vi "LinearFilter_Execute_OLD.vi"(6 "Samples":i32=3 min=1, 7 "Filter Type":T1(ring), 8 "SamplePeriod":dbl=0.02 format="%13.5f", 9 "TimeConstant":dbl=0.02 format="%13.5f", 10 "Enable":bool=TRUE, 11 "Input":dbl format="%13.5p") -> (1 "Output":dbl format="%13.5p", 3 "Out LINEAR_FILTER":T2 {"Outputs" format="%13.5g"; "Inputs" format="%13.5g"; "OutputGains" format="%13.5g"; "InputGains" format="%13.5g"})   [LabVIEW 2019, in "Trajectory_Library.lvlib"]
doc: "This is a LabVIEW \"convience\" function that combines the various subVI for a linear filter into a single subVI. This subVI creates and executes the linear filter. The filter can be dynamically enabled and disabled. When the filter is disabled, the input is transfered directly to the output. Bumpless transfer is provided when enabling the filter. Bumpless transfer is NOT provided when disabling the filter. The output value jumps directly to the current input value. The filter type and filter constants can also be changed dynamically. When the filter contstants are changed, the output may jump to the current input value when the internal buffers are reset to the current input value.\n\nInputs:\n - FilterType - An enumerated value used to select the type of filter to be cofigured. The possible values are:\n - Moving Average - Specify the \"sample\" input.\n - Low pass 1st order Butterworth filter\n - Low pass 2nd order Butterworth filter\n - High pass 1st order Butterworth filter\n - High pass 2nd order Butterworth filter\n - Input - Input value to be filtered (Required) \n - Enable - Boolean indicating filtering should be performed (Default = True)\n - TimeConstant - Filtering time constant seconds. Used for all types except Moving \n Average (Default = 0.020) \n - SamplePeriod - Execution period seconds. Used for all types except Moving Average. \n (Default = 0.020)\n - Samples - Number of samples for the moving average filter. (Default = 3)\n\nOutputs:\n - OutLinearFilter - Current value of the LinearFilter data structure.\n - Output - Current output value."
uses:
  Trajectory_Library.lvlib
  TypeDef/LINEAR_FILTER.ctl
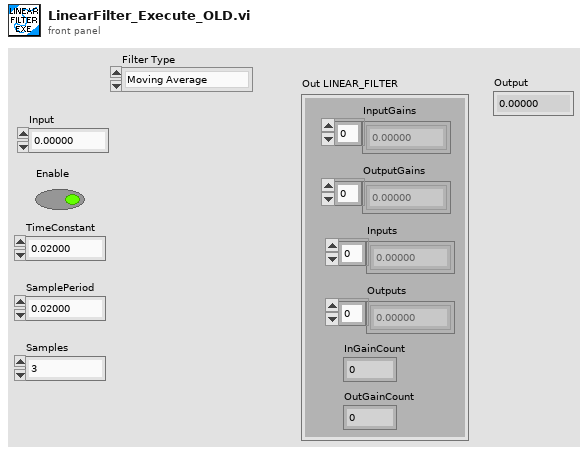
[diagram p1: front panel]
types:
  T1 = enum16{"Moving Average", "Low Pass 1st Order Butterworth", "Low Pass 2nd Order Butterworth", "High Pass 1st Order Butterworth", "High Pass 2nd Order Butterworth"}
  T2 = typedef "Trajectory_Library.lvlib/LINEAR_FILTER.ctl" = cluster{"InputGains":dbl[], "OutputGains":dbl[], "Inputs":dbl[], "Outputs":dbl[], "InGainCount":i32, "OutGainCount":i32}
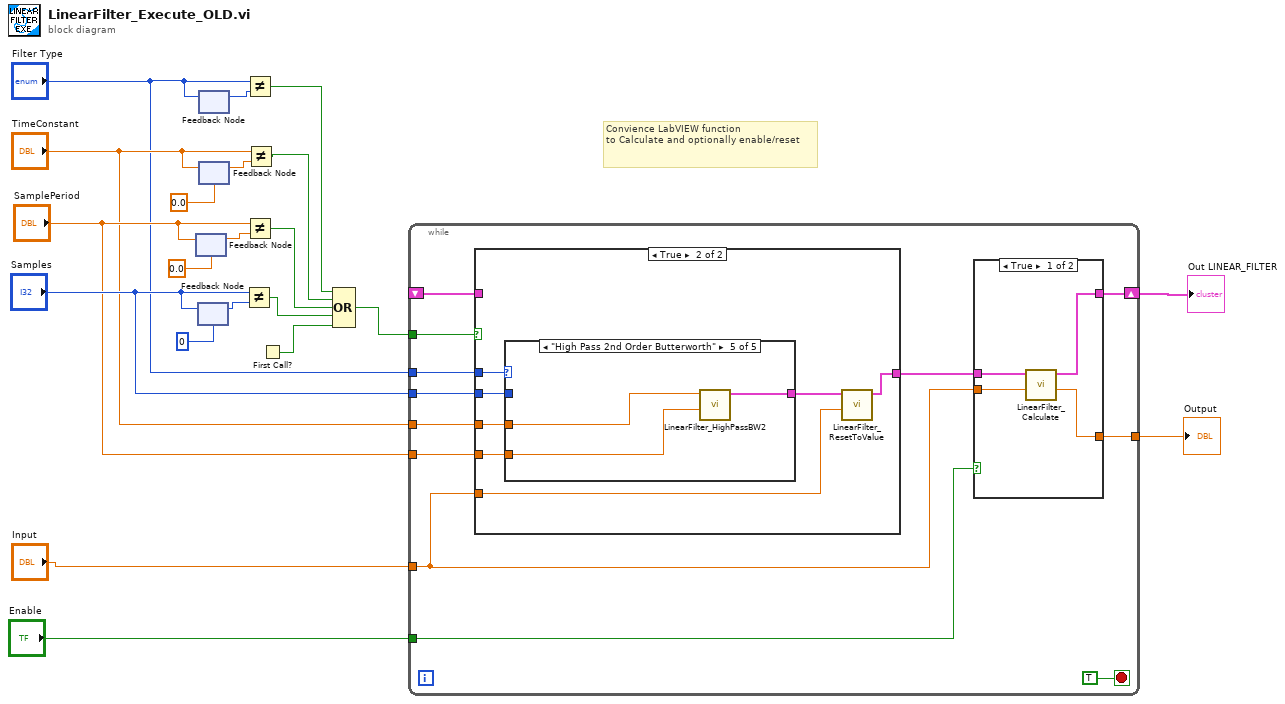
[diagram p0: block diagram]
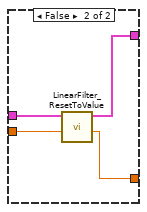
[diagram p2: hidden frame]
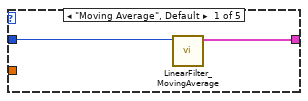
[diagram p4: hidden frame]
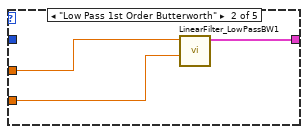
[diagram p5: hidden frame]
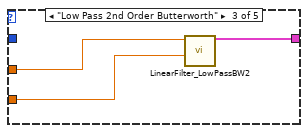
[diagram p6: hidden frame]
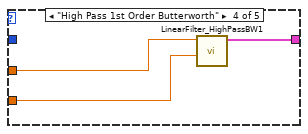
[diagram p7: hidden frame]
diagram:
  # "Convience LabVIEW function\nto Calculate and optionally enable/reset"
  n1 = feedback #1(0.0 ("SamplePeriod")) -> (w7:dbl)
  n2 = feedback-in #1("SamplePeriod") -> ()
  n3 = feedback #2(0 ("Samples")) -> (w6:i32)
  n4 = feedback-in #2("Samples") -> ()
  n5 = feedback-in #3("Filter Type") -> ()
  n6 = feedback #3() -> (w9:T1)  [unwired: 1 in]
  n7 = feedback #4(0.0 ("TimeConstant")) -> (w8:dbl)
  n8 = feedback-in #4("TimeConstant") -> ()
  n9 = Not Equal?(x="Samples", y=w6) -> (x != y?=w15:bool)
  n10 = Not Equal?(x="Filter Type", y=w9) -> (x != y?=w18:bool)
  n11 = Not Equal?(x="SamplePeriod", y=w7) -> (x != y?=w16:bool)
  n12 = Not Equal?(x="TimeConstant", y=w8) -> (x != y?=w17:bool)
  n13 = First Call?() -> (First Call?: T/F=w14:bool)
  n14 = Compound Arithmetic op=OR(w18, w17, w16, w15, w14) -> (w4:bool)
  n15 = while {
    tunnel: "Enable" -> [w33]
    tunnel: "Samples" -> [w29]
    tunnel: "SamplePeriod" -> [w28]
    tunnel: "TimeConstant" -> [w27]
    tunnel: "Filter Type" -> [w26]
    tunnel: w4 -> [w24]
    tunnel: "Input" -> [w31]
    tunnel: [w32] -> w20
    shift-right: [w25] -> w5
    shift-left: _ -> [w22]
    stop <- TRUE stop-if-true
    n16 = case shown="True" w24 {
      tunnel: w28 -> [_ w47]
      tunnel: w27 -> [_ w46]
      tunnel: w29 -> [_ w45]
      tunnel: w26 -> [_ w44]
      tunnel: w31 -> [_ w43]
      tunnel: [w41 w42] -> w30
      tunnel: w22 -> [w41 _]
      frame False {
      }
      frame True {
        n17 = case shown="\"High Pass 2nd Order Butterworth\"" w44 {
          tunnel: [w50 w51 w56 w59 w62] -> w48
          tunnel: w45 -> [w49 _ _ _ _]
          tunnel: w47 -> [_ w52 w54 w57 w60]
          tunnel: w46 -> [_ w53 w55 w58 w61]
          frame "Moving Average", Default {
            n18 = call "LinearFilter_MovingAverage.vi"("Samples"=w49) -> ("LINEAR_FILTER"=w50:T2)  [unwired: 9 in, 1 out]
          }
          frame "Low Pass 1st Order Butterworth" {
            n19 = call "LinearFilter_LowPassBW1.vi"("SamplePeriod"=w52, "TimeConstant"=w53) -> ("LINEAR_FILTER"=w51:T2)  [unwired: 9 in]
          }
          frame "Low Pass 2nd Order Butterworth" {
            n20 = call "LinearFilter_LowPassBW2.vi"("SamplePeriod"=w54, "TimeConstant"=w55) -> ("LINEAR_FILTER"=w56:T2)  [unwired: 9 in]
          }
          frame "High Pass 1st Order Butterworth" {
            n21 = call "LinearFilter_HighPassBW1.vi"("SamplePeriod"=w57, "TimeConstant"=w58) -> ("LINEAR_FILTER"=w59:T2)  [unwired: 9 in]
          }
          frame "High Pass 2nd Order Butterworth" {
            n22 = call "LinearFilter_HighPassBW2.vi"("SamplePeriod"=w60, "TimeConstant"=w61) -> ("LINEAR_FILTER"=w62:T2)  [unwired: 9 in]
          }
        }
        n23 = call "LinearFilter_ResetToValue.vi"("InputValue"=w43, "In LINEAR_FILTER"=w48) -> ("Out LINEAR_FILTER"=w42:T2)  [unwired: 9 in]
      }
    }
    n24 = case shown="True" w33 {
      tunnel: w30 -> [w37 w40]
      tunnel: [w36 w39] -> w25
      tunnel: w31 -> [w35 w38]
      tunnel: [w34 w38] -> w32
      frame True {
        n25 = call "LinearFilter_Calculate.vi"("Input"=w35, "In LINEAR_FILTER"=w37) -> ("Output"=w34:dbl, "Out LINEAR_FILTER"=w36:T2)  [unwired: 8 in]
      }
      frame False {
        n26 = call "LinearFilter_ResetToValue.vi"("InputValue"=w38, "In LINEAR_FILTER"=w40) -> ("Out LINEAR_FILTER"=w39:T2)  [unwired: 9 in]
      }
    }
  }
  "Out LINEAR_FILTER" <- w5
  "Output" <- w20
